vi "TestLogging.vi"() -> ()   [LabVIEW 2016]
uses:
  <vilib>/Rock Robotics/WPI/DriverStation/WPI_DriverStationRobotMode2.ctl
  <vilib>/Rock Robotics/Network Tables/NT Read String.vi
  <vilib>/Rock Robotics/Network Tables/NT Read Number.vi
  <vilib>/Rock Robotics/WPI/Utilities/WPI_GetSetVariantRefNum.vi
  Robot Global Data.vi
  <vilib>/Rock Robotics/Network Tables/NT Write Number.vi
  <vilib>/Rock Robotics/Network Tables/NT Write String.vi
panel:
  in  "Diagnostic":string
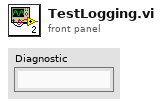
[diagram p1: front panel]
types:
  T1 = enum16{"open", "replace", "create", "open or create", "replace or create", "replace or create with confirmation"}
  T2 = typedef "WPI_DriverStationRobotMode2.ctl" = enum16{"Autonomous Disabled", "Autonomous Enabled", "Teleop Disabled", "Teleop Enabled", "Disconnected", "Finish", "Test Disabled", "Test Enabled", "Emergency Stopped"}
  T3 = typedef "WPI_JoystickDevRef.ctl" = cluster{"Device":T4}
  T4 = typedef "WPI_JoystickDeviceEnum.ctl" = enum16{"USB 0", "USB 1", "USB 2", "USB 3", "USB 4", "USB 5"}
  T5 = typedef "Z900_navX_Flags_OpStatusTypeDef.ctl" = u8
  T6 = typedef "Z900_navX_Flags_CalibrationStatusTypeDef.ctl" = u8
  T7 = cluster{"Update Rate Hz":u8, "Accelerometer Full-Scale Range":u8, "Gyro Full-Scale Range":u16, "OP Status":T5, "Calibration Status":T6, "Sensor Status":cluster{"MOVING":bool, "YAW_STABLE":bool, "MAG_DISTURBANCE":bool, "ALTITUDE_VALID":bool, "SEALEVEL_PRESS_SET":bool, "FUSED_HEADING_VALID":bool}, "Self Test Status":cluster{"Gyro Passed":bool, "Accel Passed":bool, "Mag Passed":bool, "Baro Passed":bool, "Complete":bool}}
  T8 = cluster{"Yaw":dbl, "Roll":dbl, "Pitch":dbl, "Heading":dbl, "Fused Heading":dbl}
  T9 = cluster{"LinearAcceleration X":dbl, "LinearAcceleration Y":dbl, "LinearAcceleration Z":dbl}
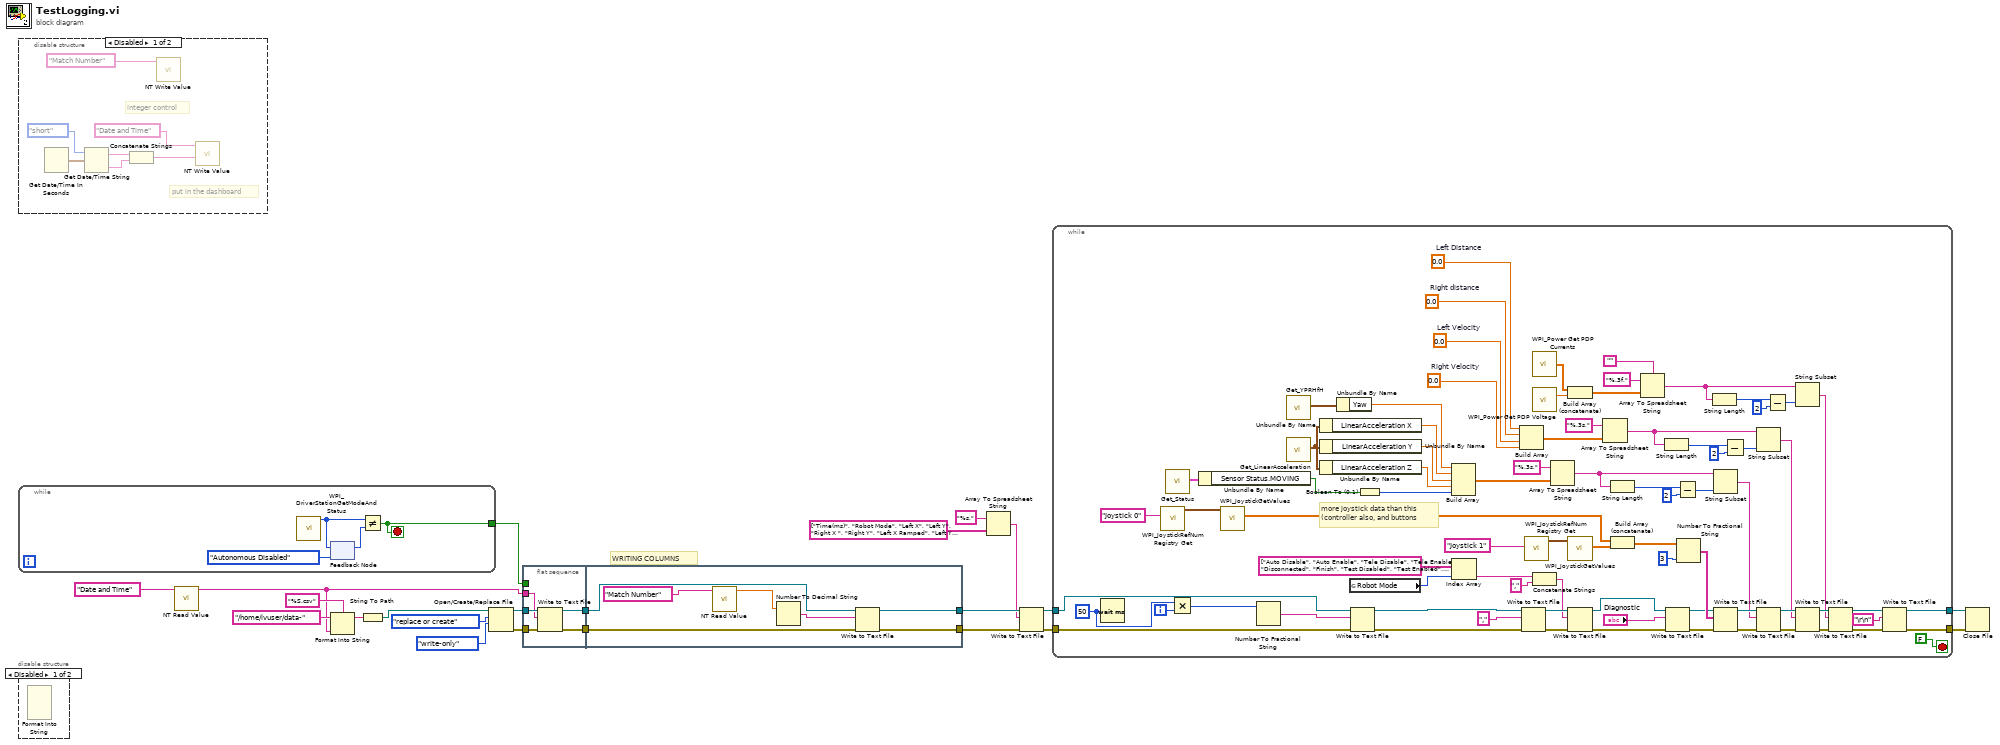
[diagram p0: block diagram]
diagram:
  # "WRITING COLUMNS"
  n1 = disable-structure shown="Disabled" {
    frame Disabled {
      # "integer control"
      # "put in the dashboard"
      n2 = Get Date/Time In Seconds() -> (seconds since 1Jan1904=w29:timestamp)
      n3 = Get Date/Time String(date format (0)=enum16{"short", "long", "abbreviated"}."short", seconds (now)=w29) -> (date string=w26:string, time string=w27:string)  [unwired: 1 in]
      n4 = Concatenate Strings(w26, w27) -> (w25:string)
      n5 = call-poly <vilib>:"NT Write Value.vi"("Name"="Match Number") -> ()  [unwired: 10 in, 1 out]
      n6 = call-poly <vilib>:"NT Write Value.vi"("String"=w25, "Name"="Date and Time") -> ()  [unwired: 9 in, 1 out]
    }
    frame Enabled {
    }
  }
  n7 = while {
    tunnel: [w30] -> w17
    stop <- w30 stop-if-true
    n8 = call <vilib>:"WPI_DriverStationGetModeAndStatus.vi"() -> ("Robot Mode"=w31:T2)  [unwired: 10 in, 1 out]
    n9 = feedback #1(WPI_DriverStationRobotMode2."Autonomous Disabled" ("Robot Mode")) -> (w32:T2)
    n10 = feedback-in #1(w31) -> ()
    n11 = Not Equal?(x=w31, y=w32) -> (x != y?=w30:bool)
  }
  n12 = disable-structure shown="Disabled" {
    frame Disabled {
      n13 = Format Into String() -> ()  [unwired: 6 in, 2 out]
    }
    frame Enabled {
    }
  }
  n14 = call-poly <vilib>:"NT Read Value.vi"("Name"="Date and Time") -> ("String"=w9:string)  [unwired: 9 in, 1 out]
  n15 = Format Into String(format string="%S.csv", initial string="/home/lvuser/data-", w9) -> (resulting string=w18:string)  [unwired: 1 in, 1 out]
  n16 = String To Path(string=w18) -> (path=w11:path)
  n17 = Open/Create/Replace File(file path (use dialog)=w11, operation (0:open)=T1."replace or create", access (0:read/write)=enum16{"read/write", "read-only", "write-only"}."write-only") -> (refnum out=w16:refnum<file>, error out=w15:errorcluster)  [unwired: 3 in, 1 out]
  n18 = flat-sequence {
    tunnel: w17 -> [_]
    tunnel: w16 -> [w38]
    tunnel: w15 -> [w37]
    tunnel: [w36] -> w14
    tunnel: [w35] -> w13
    tunnel: w9 -> [w34]
    tunnel: w14 -> [w44]
    tunnel: w13 -> [w43]
    tunnel: [w40] -> w8
    tunnel: [w39] -> w7
    frame #0 {
      n19 = Write to Text File(file (use dialog)=w38, text=w34, error in=w37) -> (refnum out=w35:refnum<file>, error out=w36:errorcluster)  [unwired: 1 in, 1 out]
    }
    frame #1 {
      n20 = call-poly <vilib>:"NT Read Value.vi"("Name"="Match Number") -> ("Numeric"=w42:dbl)  [unwired: 9 in, 1 out]
      n21 = Number To Decimal String(number=w42) -> (decimal integer string=w41:string)  [unwired: 1 in]
      n22 = Write to Text File(file (use dialog)=w43, text=w41, error in=w44) -> (refnum out=w40:refnum<file>, error out=w39:errorcluster)  [unwired: 1 in, 1 out]
    }
  }
  n23 = Array To Spreadsheet String(array=string[] ["Time(ms)", "Robot Mode", "Left X", "Left Y", "Right X ", "Right Y", "Left X Ramped", "Left Y Ramped", "Right X Ramped", "Right Y Ramped", "Diagnostic Messages", "Yaw", "X, Y, Z axis acceleration", "Moving?", "Left Distance", "Right Distance", "Left Velocity", "Right Velocity", "Voltage", "Channel 0 current", "Channel 1 current", "Channel 2 current", "Channel 3 current", "Channel 4 current", "Channel 5 current", "Channel 6 current", "Channel 7 current", "Channel 8 current", "Channel 9 current"], 3:"%s," ("delimiter (Tab)")) -> (spreadsheet string=w2:string)  [unwired: 1 in]
  n24 = Write to Text File(file (use dialog)=w8, text=w2, error in=w7) -> (refnum out=w5:refnum<file>, error out=w6:errorcluster)  [unwired: 1 in, 1 out]
  n25 = while {
    tunnel: [w115] -> w21
    tunnel: w5 -> [w98]
    tunnel: w6 -> [w97]
    tunnel: [w72] -> w1
    i -> [w123]
    stop <- FALSE stop-if-true
    w95 = 0.0  # Right distance
    w96 = 0.0  # Left Distance
    w93 = 0.0  # Right Velocity
    w94 = 0.0  # Left Velocity
    w124 = u32 50 ("milliseconds to wait")
    # "more joystick data than this\n(controller also, and buttons"
    n26 = Wait (ms)(milliseconds to wait=w124) -> ()  [unwired: 1 out]
    n27 = call <vilib>:"WPI_JoystickRefNum Registry Get.vi"("refnum name"="Joystick 0") -> ("JoystickDevRef"=w114:T3)  [unwired: 9 in, 1 out]
    n28 = call <userlib>:"Get_Status.vi"() -> ("Status"=w75:T7)  [unwired: 11 in]
    n29 = Multiply(x=w124, y=w123) -> (x*y=w122:u32)
    n30 = Unbundle By Name(w75) -> ("Sensor Status.MOVING"=w77:bool)
    n31 = call <vilib>:"WPI_JoystickGetValues.vi"("JoystickDevRef"=w114) -> ("Axes"=w110:dbl[])  [unwired: 6 in, 4 out]
    n32 = Number To Fractional String(number=w122) -> (F-format string=w104:string)  [unwired: 3 in]
    n33 = call <userlib>:"Get_YPRHfH.vi"() -> ("YRPHfH"=w88:T8)  [unwired: 11 in]
    n34 = call <userlib>:"Get_LinearAcceleration.vi"() -> ("Linear Acceleration"=w87:T9)  [unwired: 11 in]
    n35 = Unbundle By Name(w87) -> ("LinearAcceleration X"=w84:dbl)
    n36 = Unbundle By Name(w87) -> ("LinearAcceleration Y"=w85:dbl)
    n37 = Unbundle By Name(w87) -> ("LinearAcceleration Z"=w83:dbl)
    n38 = Unbundle By Name(w88) -> ("Yaw"=w86:dbl)
    n39 = global read "Robot Global Data.vi" "Robot Mode"() -> (w71:T2)
    n40 = Write to Text File(file (use dialog)=w98, text=w104, error in=w97) -> (refnum out=w121:refnum<file>, error out=w117:errorcluster)  [unwired: 1 in, 1 out]
    n41 = Boolean To (0,1)(Boolean=w77) -> (0, 1=w76:i16)
    n42 = Build Array(w86, w84, w85, w83, w76) -> (w70:dbl[])
    n43 = Index Array(array=string[] ["Auto Disable", "Auto Enable", "Tele Disable", "Tele Enable", "Disconnected", "Finish", "Test Disabled", "Test Enabled", "Emergency Stopped"] ("Strings []"), index=w71) -> (element=w101:string)
    n44 = Build Array(w96, w95, w94, w93) -> (w92:dbl[])
    n45 = Write to Text File(file (use dialog)=w121, text=",", error in=w117) -> (refnum out=w100:refnum<file>, error out=w99:errorcluster)  [unwired: 1 in, 1 out]
    n46 = call <vilib>:"WPI_JoystickRefNum Registry Get.vi"("refnum name"="Joystick 1") -> ("JoystickDevRef"=w112:T3)  [unwired: 9 in, 1 out]
    n47 = call <vilib>:"WPI_Power Get PDP Currents.vi"() -> ("all currents (A)"=w118:dbl[])  [unwired: 13 in, 2 out]
    n48 = call <vilib>:"WPI_Power Get PDP Voltage.vi"() -> ("voltage (V)"=w105:dbl)  [unwired: 14 in, 1 out]
    n49 = Concatenate Strings(w101, "," ("string")) -> (w62:string)
    n50 = Array To Spreadsheet String(array=w70, 3:"%.3s," ("spreadsheet string")) -> (spreadsheet string=w65:string)  [unwired: 1 in]
    n51 = Build Array (concatenate)(w118, w105) -> (w69:dbl[])
    n52 = call <vilib>:"WPI_JoystickGetValues.vi"("JoystickDevRef"=w112) -> ("Axes"=w109:dbl[])  [unwired: 6 in, 4 out]
    n53 = Write to Text File(file (use dialog)=w100, text=w62, error in=w99) -> (refnum out=w61:refnum<file>, error out=w59:errorcluster)  [unwired: 1 in, 1 out]
    n54 = Array To Spreadsheet String(array=w92, 3:"%.3s," ("delimiter (Tab)")) -> (spreadsheet string=w47:string)  [unwired: 1 in]
    n55 = String Length(string=w65) -> (length=w68:i32)
    n56 = Build Array (concatenate)(w110, w109) -> (w108:dbl[])
    n57 = Array To Spreadsheet String(delimiter (Tab)="", array=w69, 3:"%.3f," ("format string")) -> (spreadsheet string=w54:string)
    n58 = String Length(string=w47) -> (length=w49:i32)
    n59 = Write to Text File(file (use dialog)=w61, text="Diagnostic", error in=w59) -> (refnum out=w60:refnum<file>, error out=w58:errorcluster)  [unwired: 1 in, 1 out]
    n60 = Subtract(x=w68, y=2) -> (x-y=w66:i32)
    n61 = Number To Fractional String(number=w108, precision (6)=i16 3) -> (F-format string=w63:string[])  [unwired: 2 in]
    n62 = String Length(string=w54) -> (length=w55:i32)
    n63 = String Subset(string=w65, length (rest)=w66) -> (substring=w53:string)  [unwired: 1 in]
    n64 = Write to Text File(file (use dialog)=w60, text=w63, error in=w58) -> (refnum out=w82:refnum<file>, error out=w79:errorcluster)  [unwired: 1 in, 1 out]
    n65 = Subtract(x=w49, y=2) -> (x-y=w51:i32)
    n66 = String Subset(string=w47, length (rest)=w51) -> (substring=w46:string)  [unwired: 1 in]
    n67 = Write to Text File(file (use dialog)=w82, text=w53, error in=w79) -> (refnum out=w81:refnum<file>, error out=w80:errorcluster)  [unwired: 1 in, 1 out]
    n68 = Subtract(x=w55, y=2) -> (x-y=w57:i32)
    n69 = String Subset(string=w54, length (rest)=w57) -> (substring=w48:string)  [unwired: 1 in]
    n70 = Write to Text File(file (use dialog)=w81, text=w46, error in=w80) -> (refnum out=w90:refnum<file>, error out=w89:errorcluster)  [unwired: 1 in, 1 out]
    n71 = Write to Text File(file (use dialog)=w90, text=w48, error in=w89) -> (refnum out=w74:refnum<file>, error out=w73:errorcluster)  [unwired: 1 in, 1 out]
    n72 = Write to Text File(file (use dialog)=w74, text="\r\n", error in=w73) -> (refnum out=w115:refnum<file>, error out=w72:errorcluster)  [unwired: 1 in, 1 out]
  }
  n73 = Close File(refnum=w21, error in=w1) -> ()  [unwired: 2 out]
